vi "wrap.TableSetNumber.vi"(0 "class.GLue in":refnum<class "class.GLue.lvclass">, 2 "Number":dbl, 11 "error in (no error)":errorcluster, 13 "Name":string) -> (4 "class.GLue out":refnum<class "class.GLue.lvclass">, 15 "error out":errorcluster)   [LabVIEW 2014, in "GLue.lvlib" / "class.GLue.lvclass"]
uses:
  class.GLue.lvclass
  class.GLue.lvclass/class.GLue.ctl
  Resources/GLue.dll
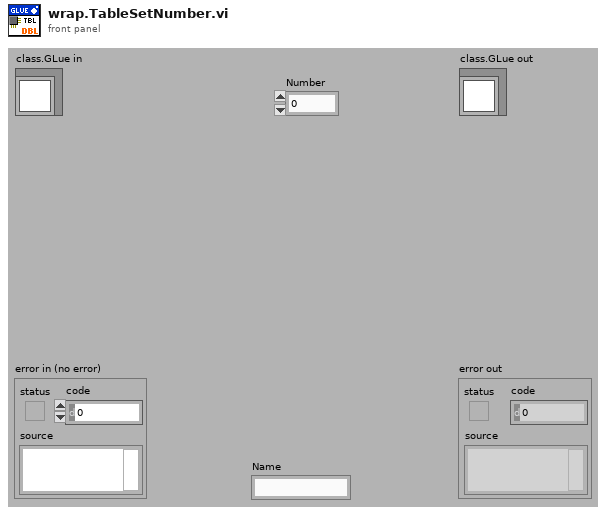
[diagram p1: front panel]
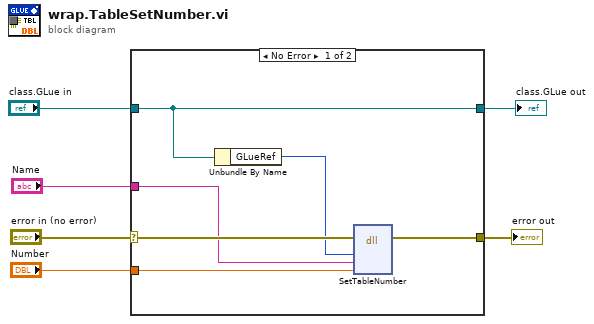
[diagram p0: block diagram]
diagram:
  n1 = case shown="No Error" "error in (no error)" {
    selector: "error in (no error)" -> [w11 w14]
    tunnel: [w10 w14] -> w5
    tunnel: [w12 w13] -> w3
    tunnel: "class.GLue in" -> [w12 w13]
    tunnel: "Name" -> [w8 _]
    tunnel: "Number" -> [w7 _]
    frame No Error {
      n2 = Unbundle By Name(w12) -> ("GLueRef"=w9:i64)
      n3 = dll-call lib="C:/Users/Antonie/Documents/work/glue/trunk/Resources/GLue.dll" fn="SetTableNumber"(error in=w11, "MLua"=w9, "Name"=w8, "Number"=w7) -> (error out=w10:errorcluster)  [unwired: 6 in, 1 out]
    }
    frame Error {
    }
  }
  "error out" <- w5
  "class.GLue out" <- w3
